vi "Host_Main.vi"() -> ()   [LabVIEW 2016]
uses:
  Typedefs/IO Lines State.ctl
  Typedefs/IO Lines Enable.ctl
  Typedefs/Truncate Waveform Settings.ctl
  Typedefs/Monitor Data Operation.ctl
  Typedefs/Host Cluster.ctl
  Typedefs/LV2G Operation.ctl
  <vilib>/NI/AMC/Read Termination Message.vi
  <vilib>/NI/AMC/Create Single Message.vi
  <vilib>/NI/AMC/Update Message Routing Info.vi
  <vilib>/NI/AMC/Globals.vi
  <vilib>/NI/AMC/Send Message.vi
  <vilib>/NI/AMC/AMC.lvlib
panel:
  in  "Tab Control":enum32{"Pattern", "Instruction"}(tab)
  out "Read Digital Waveform Graph":digitalwaveform(graph)
  in  "Truncate Waveform Settings":T1 {"End Idle Time(us)" format="%#.2f"; "Start Idle Time(us)" format="%#.2f"}
  out "Elapsed Time(ms)":u32 max=42
  in  "Monitor Time(ms)":u32 max=42000
  in  "IO Lines Read  Enable":T2={"Enable"=[FALSE, FALSE, FALSE, FALSE, FALSE, FALSE, FALSE, FALSE, FALSE, FALSE, FALSE, FALSE, FALSE, FALSE, FALSE, FALSE, FALSE, FALSE, FALSE, FALSE, FALSE, FALSE, FALSE, FALSE, FALSE, FALSE, FALSE, FALSE, FALSE, FALSE, FALSE, FALSE]}
  in  "Exit":bool
  in  "IO Lines Write  Enable":T2={"Enable"=[FALSE, FALSE, FALSE, FALSE, FALSE, FALSE, FALSE, FALSE, FALSE, FALSE, FALSE, FALSE, FALSE, FALSE, FALSE, FALSE, FALSE, FALSE, FALSE, FALSE, FALSE, FALSE, FALSE, FALSE, FALSE, FALSE, FALSE, FALSE, FALSE, FALSE, FALSE, FALSE]}
  in  "Monitoring":bool
  in  "Write Pattern":bool
  out "Write Digital Waveform Graph":digitalwaveform(graph)
  in  "IO Lines Pattteen":T3[](array[typedef]) {"Duration (us)" min=0.005 max=42550000.0 step=0.005 format="%#.3f"}
  # "Generator Settings"
  # "Monitor Settings"
  # "Duration(us)"
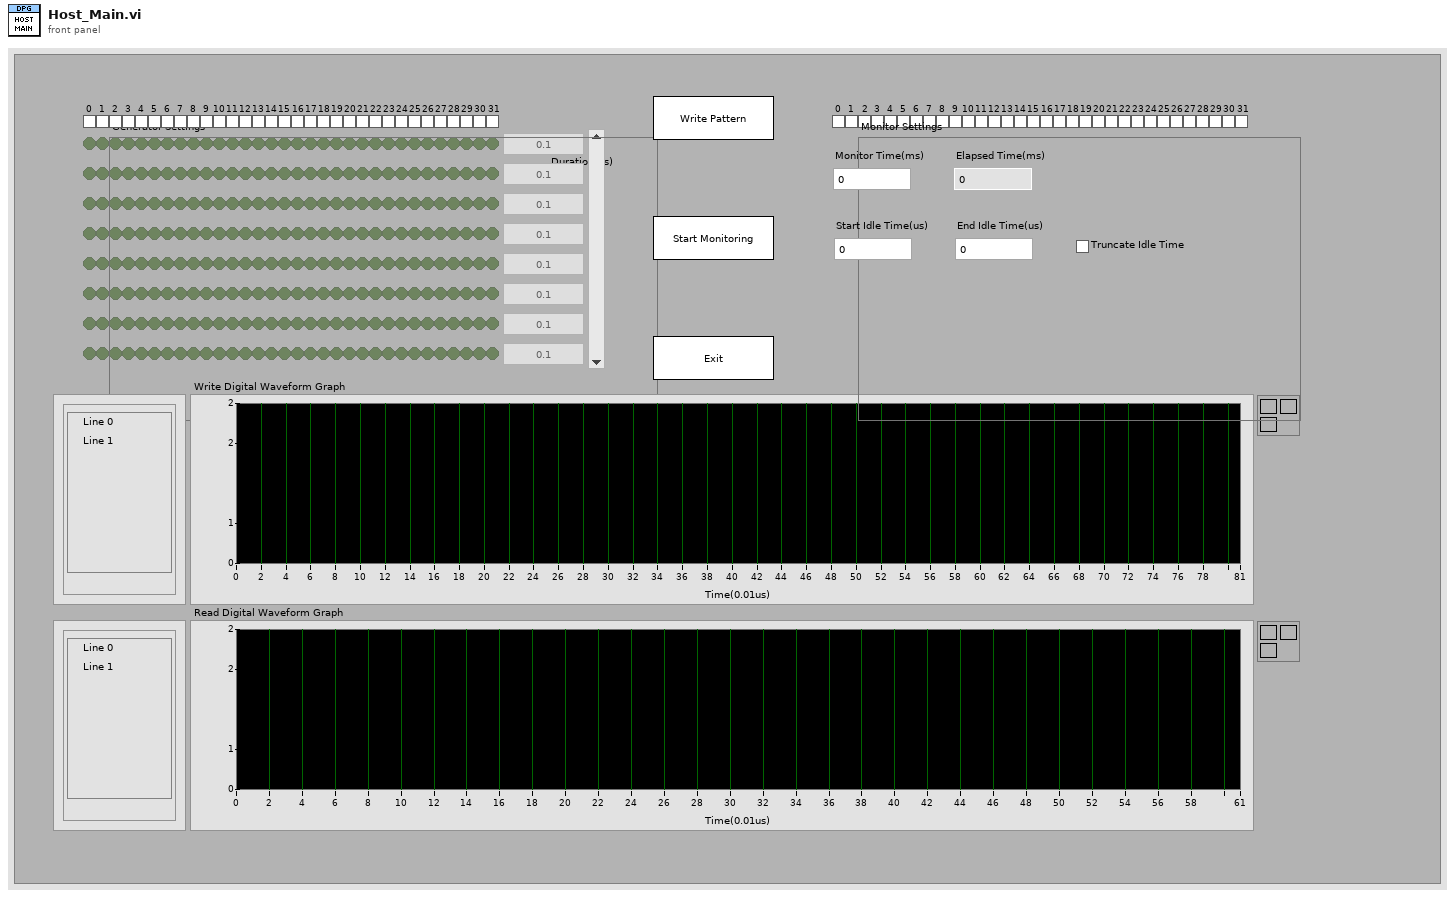
[diagram p1: front panel]
types:
  T1 = typedef "Truncate Waveform Settings.ctl" = cluster{"Truncate Idle Time":bool, "Start Idle Time(us)":dbl, "End Idle Time(us)":dbl}
  T2 = typedef "IO Lines Enable.ctl" = cluster{"Enable":bool[]}
  T3 = typedef "IO Lines State.ctl" = cluster{"State":bool[], "Duration (us)":dbl}
  T4 = typedef "AMC.lvlib/Message Queue.ctl" = refnum<queue>
  T5 = typedef "Monitor Data Operation.ctl" = enum16{"Obtain", "Enqueue", "Read Elements", "Flush", "Release", "Read Last Element"}
  T6 = typedef "Monitor Data Element.ctl" = cluster{"Pin Data":u32, "Transition ":u32}
  T7 = typedef "Host Cluster.ctl" = cluster{"Monitor Enable?":bool, "Start Time(ms)":u32}
  T8 = typedef "LV2G Operation.ctl" = enum16{"Initialize", "Set", "Get", "Close"}
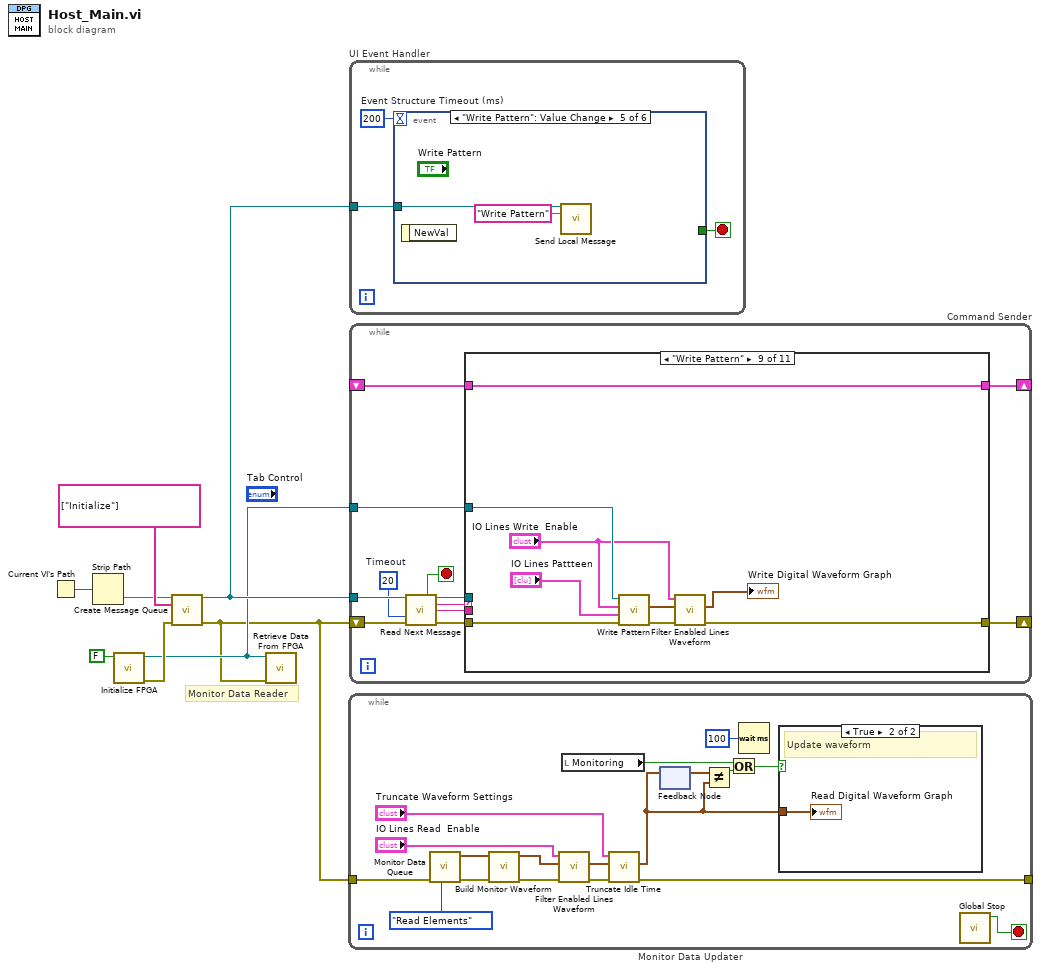
[diagram p0: block diagram]
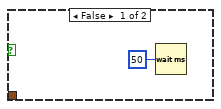
[diagram p2: hidden frame]
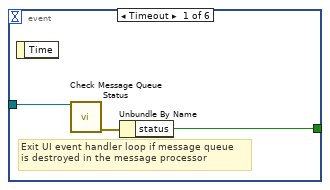
[diagram p3: hidden frame]
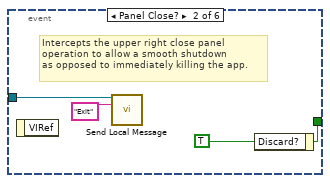
[diagram p4: hidden frame]
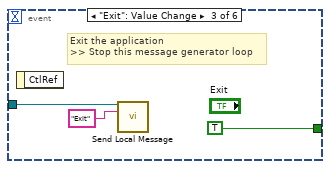
[diagram p5: hidden frame]
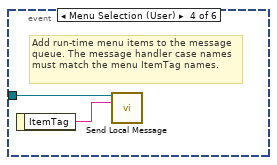
[diagram p6: hidden frame]
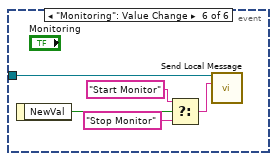
[diagram p7: hidden frame]
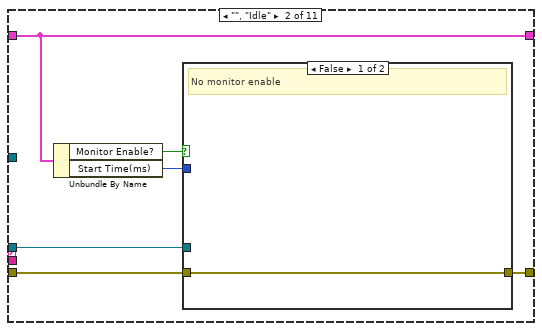
[diagram p9: hidden frame]
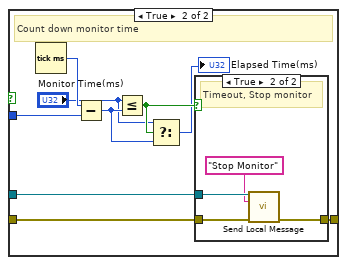
[diagram p10: hidden frame]
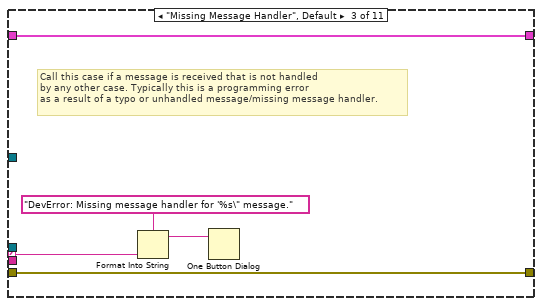
[diagram p12: hidden frame]
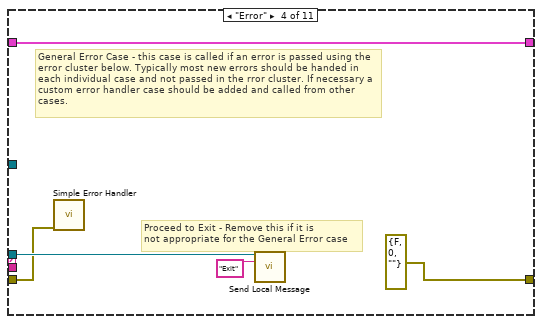
[diagram p13: hidden frame]
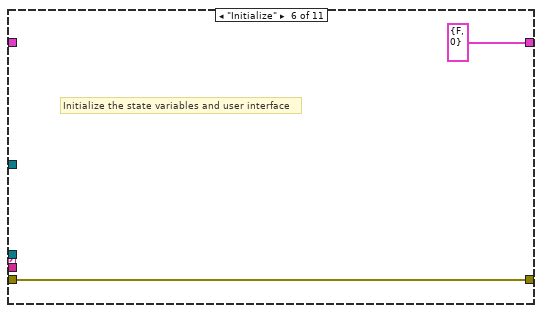
[diagram p15: hidden frame]
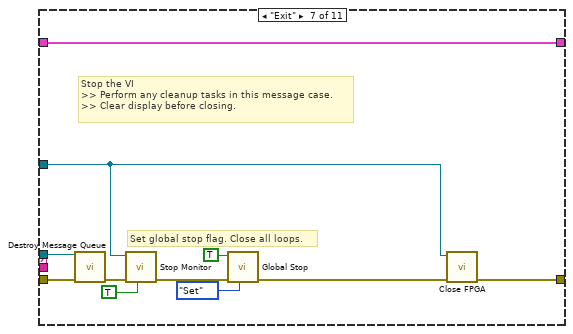
[diagram p16: hidden frame]
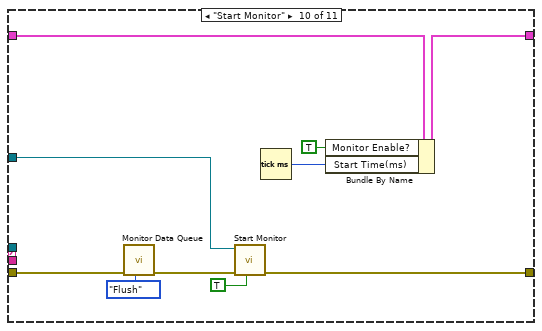
[diagram p18: hidden frame]
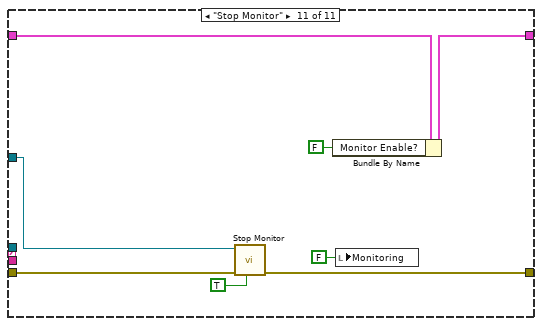
[diagram p19: hidden frame]
diagram:
  # "Monitor Data Reader"
  n1 = Current VI's Path() -> (path=w5:path)
  n2 = Strip Path(path=w5) -> (name=w7:string)  [unwired: 1 out]
  n3 = call "Initialize FPGA.vi"("Simulation?"=FALSE) -> ("error out"=w4:errorcluster, "FPGA VI Reference"=w3:refnum<k20>)  [unwired: 9 in]
  n4 = call <vilib>:"Create Message Queue.vi"("message queue name"=w7, "initial message names"=string[] ["Initialize"], "error in"=w4) -> ("message queue out"=w6:T4, "error out"=w2:errorcluster)  [unwired: 11 in]
  n5 = call "Retrieve Data From FPGA.vi"("error in (no error)"=w2, "FPGA VI Reference In"=w3) -> ()  [unwired: 9 in, 1 out]
  n6 = while "Monitor Data Updater" {
    tunnel: w2 -> [w26]
    tunnel: [w15] -> _
    stop <- w24 stop-if-true
    n7 = call "Monitor Data Queue.vi"("Queue Function"=Monitor_Data_Operation."Read Elements", "error in (no error)"=w26) -> ("error out"=w23:errorcluster, "Queue Elements"=w12:T6[])  [unwired: 6 in, 2 out]
    n8 = call "Build Monitor Waveform.vi"("error in (no error)"=w23, "Queue Elements"=w12) -> ("error out"=w22:errorcluster, "Digital Data Table"=w10:digitaldata)  [unwired: 8 in]
    n9 = call "Filter Enabled Lines Waveform.vi"("error in (no error)"=w22, "Pattern Digital Data"=w10, "IO Lines Enable"="IO Lines Read  Enable") -> ("error out"=w16:errorcluster, "Digital Waveform"=w14:digitalwaveform)  [unwired: 7 in]
    n10 = local read "Monitoring"() -> (w20:bool)
    n11 = call "Truncate Idle Time.vi"("error in (no error)"=w16, "Digital Waveform"=w14, "Truncate Waveform Settings"="Truncate Waveform Settings") -> ("error out"=w15:errorcluster, "Digital Waveform out"=w11:digitalwaveform)  [unwired: 7 in]
    n12 = feedback-in #1(w11) -> ()
    n13 = feedback #1() -> (w19:digitalwaveform)  [unwired: 1 in]
    n14 = Not Equal?(x=w19, y=w11) -> (x != y?=w17:bool)
    n15 = Or(x=w20, y=w17) -> (x .or. y?=w18:bool)
    n16 = Wait (ms)(milliseconds to wait=u32 100) -> ()  [unwired: 1 out]
    n17 = case shown="True" w18 {
      tunnel: w11 -> [_ w28]
      frame False {
        n18 = Wait (ms)(milliseconds to wait=u32 50) -> ()  [unwired: 1 out]
      }
      frame True {
        # "Update waveform"
        "Read Digital Waveform Graph" <- w28
      }
    }
    n19 = call "Global Stop.vi"() -> ("Stop? out"=w24:bool)  [unwired: 10 in, 1 out]
  }
  n20 = while "UI Event Handler" {
    tunnel: w6 -> [w29]
    stop <- w30 stop-if-true
    w31 = 200  # Event Structure Timeout (ms)
    n21 = event shown="[4] \"Write Pattern\": Value Change" {
      selector: _ -> [_ _ _ _ _ _]
      dyn-events: _ -> [_ _ _ _ _ _]
      timeout: w31 -> [_ _ _ _ _ _]
      tunnel: [w32 w37 TRUE ("Discard?") _ _ _] -> w30
      tunnel: w29 -> [w33 w35 w38 w41 w44 w49]
      event Timeout {
        # "Exit UI event handler loop if message queue\nis destroyed in the message processor"
        n22 = event-data() -> ()  [unwired: 2 out]
        n23 = call <vilib>:"Check Message Queue Status.vi"("message queue in"=w33) -> ("error out"=w34:errorcluster)  [unwired: 10 in, 4 out]
        n24 = Unbundle By Name(w34) -> ("status"=w32:bool)
      }
      event Panel Close? {
        w37 = TRUE ("Discard?")
        # "Intercepts the upper right close panel\noperation to allow a smooth shutdown\nas opposed to immediately killing the app."
        n25 = event-data() -> ()  [unwired: 2 out]
        n26 = call <vilib>:"Send Local Message.vi"("message queue in"=w35, "message name"="Exit") -> ()  [unwired: 11 in, 3 out]
        n27 = event-data("Discard?"=w37) -> ()  [unwired: 1 in, 1 out]
      }
      event "Exit": Value Change {
        # "Exit the application\n>> Stop this message generator loop"
        n28 = event-data() -> ()  [unwired: 2 out]
        n29 = call <vilib>:"Send Local Message.vi"("message queue in"=w38, "message name"="Exit") -> ()  [unwired: 11 in, 3 out]
      }
      event Menu Selection (User) {
        # "Add run-time menu items to the message\nqueue. The message handler case names must match the menu ItemTag names."
        n30 = event-data() -> ("ItemTag"=w42:string)  [unwired: 1 out]
        n31 = call <vilib>:"Send Local Message.vi"("message queue in"=w41, "message name"=w42) -> ()  [unwired: 11 in, 3 out]
      }
      event "Write Pattern": Value Change {
        n32 = event-data() -> ()  [unwired: 2 out]
        n33 = call <vilib>:"Send Local Message.vi"("message queue in"=w44, "message name"="Write Pattern") -> ()  [unwired: 11 in, 3 out]
      }
      event "Monitoring": Value Change {
        n34 = event-data() -> ("NewVal"=w47:bool)  [unwired: 1 out]
        n35 = Select(t="Start Monitor" ("message name"), s=w47, f="Stop Monitor") -> (s? t:f=w46:string)
        n36 = call <vilib>:"Send Local Message.vi"("message queue in"=w49, "message name"=w46) -> ()  [unwired: 11 in, 3 out]
      }
    }
  }
  n37 = while "Command Sender" {
    shift-left: w2 -> [w55]
    shift-right: [w59] -> _
    tunnel: w6 -> [w56]
    shift-left: _ -> [w61]
    shift-right: [w60] -> _
    tunnel: w3 -> [w50]
    stop <- w58 stop-if-true
    w51 = 20  # Timeout
    n38 = call <vilib>:"Read Next Message.vi"("message queue in"=w56, "timeout (1 ms)"=w51, "error in"=w55) -> ("exit process?"=w58:bool, "message queue out"=w57:T4, "message name"=w53:string, "message value"=w52:string, "error out"=w54:errorcluster)  [unwired: 5 in, 3 out]
    n39 = case shown="\"Write Pattern\"" w53 {
      selector: w53 -> [_ _ w87 _ _ _ _ _ _ _ _]
      tunnel: [w63 w69 w89 w94 w96 T7 {"Monitor Enable?"=FALSE, "Start Time(ms)"=0} ("state variables") w109 w111 w120 w123 w132] -> w60
      tunnel: w61 -> [w63 w69 w89 w94 w96 _ w109 w111 w120 w130 w138]
      tunnel: w57 -> [_ w66 _ w92 _ _ w107 _ _ _ _]
      tunnel: w54 -> [w62 w65 w88 w90 w95 w98 w108 w110 w117 w126 w137]
      tunnel: [w62 w64 w88 errorcluster {"status"=FALSE, "code"=0, "source"=""} ("error out") w95 w98 w99 w110 w112 w129 w136] -> w59
      tunnel: w52 -> [_ _ _ _ _ _ _ _ _ _ _]
      tunnel: w50 -> [_ _ _ _ _ _ w101 _ w119 w127 w134]
      frame "---------- Framework Operations ----------" {
        # "Dummy case to add a seperator in the Case Structure menu"
      }
      frame "", "Idle" {
        n40 = Unbundle By Name(w69) -> ("Monitor Enable?"=w68:bool, "Start Time(ms)"=w67:u32)
        n41 = case shown="False" w68 {
          tunnel: w67 -> [_ w78]
          tunnel: w66 -> [_ w77]
          tunnel: w65 -> [w70 w76]
          tunnel: [w70 w75] -> w64
          frame False {
            # "No monitor enable"
          }
          frame True {
            # "Count down monitor time"
            n42 = Tick Count (ms)() -> (millisecond timer value=w79:u32)
            n43 = Subtract(x=w79, y=w78) -> (x-y=w72:u32)
            n44 = Less Or Equal?(x="Monitor Time(ms)", y=w72) -> (x <= y?=w74:bool)
            n45 = Select(t="Monitor Time(ms)", s=w74, f=w72) -> (s? t:f=→"Elapsed Time(ms)":u32)
            n46 = case shown="True" w74 {
              tunnel: w77 -> [_ w84]
              tunnel: w76 -> [w80 w83]
              tunnel: [w80 w82] -> w75
              frame False {
                # "Continue"
              }
              frame True {
                # "Timeout, Stop monitor"
                n47 = call <vilib>:"Send Local Message.vi"("message queue in"=w84, "message name"="Stop Monitor", "error in"=w83) -> ("error out"=w82:errorcluster)  [unwired: 10 in, 2 out]
              }
            }
          }
        }
      }
      frame "Missing Message Handler", Default {
        # "Call this case if a message is received that is not handled \nby any other case. Typically this is a programming error\nas a result of a typo or unhandled message/missing message handler."
        n48 = Format Into String(format string="DevError: Missing message handler for '%s\" message." ("message"), w87) -> (resulting string=w85:string)  [unwired: 2 in, 1 out]
        n49 = One Button Dialog(message=w85) -> ()  [unwired: 2 out]
      }
      frame "Error" {
        # "Proceed to Exit - Remove this if it is\nnot appropriate for the General Error case"
        # "General Error Case - this case is called if an error is passed using the error cluster below. Typically most new errors should be handed in each individual case and not passed in the rror cluster. If necessary a custom error handler case should be added and called from other cases."
        n50 = call <vilib>:"Simple Error Handler.vi"("error in (no error)"=w90) -> ()  [unwired: 1 in, 8 out]
        n51 = call <vilib>:"Send Local Message.vi"("message queue in"=w92, "message name"="Exit") -> ()  [unwired: 11 in, 3 out]
      }
      frame "---------- Generic Operations ----------" {
        # "Dummy case to add a seperator in the Case Structure menu"
      }
      frame "Initialize" {
        # "Initialize the state variables and user interface"
      }
      frame "Exit" {
        # "Set global stop flag. Close all loops."
        # "Stop the VI\n>> Perform any cleanup tasks in this message case.\n>> Clear display before closing."
        n52 = call <vilib>:"Destroy Message Queue.vi"("message queue in"=w107, "error in"=w108) -> ("error out"=w104:errorcluster)  [unwired: 11 in, 2 out]
        n53 = call "Stop Monitor.vi"("Write to FPGA(T)"=TRUE, "error in (no error)"=w104, "FPGA VI Reference In"=w101) -> ("error out"=w103:errorcluster)  [unwired: 7 in, 1 out]
        n54 = call "Global Stop.vi"("Stop Operation (Get)"=LV2G_Operation."Set", "error in (no error)"=w103, "Stop?"=TRUE) -> ("error out"=w100:errorcluster)  [unwired: 7 in, 1 out]
        n55 = call "Close FPGA.vi"("error in (no error)"=w100, "Refnum in"=w101) -> ("error out"=w99:errorcluster)  [unwired: 9 in]
      }
      frame "---------- Application Operations ----------" {
        # "Dummy case to add a seperator in the Case Structure menu"
      }
      frame "Write Pattern" {
        n56 = call "Write Pattern.vi"("error in (no error)"=w117, "IO Lines Pattteen"="IO Lines Pattteen", "IO Lines Enable"="IO Lines Write  Enable", "Refnum in"=w119) -> ("error out"=w115:errorcluster, "Pattern Digital Data"=w116:digitaldata)  [unwired: 5 in, 1 out]
        n57 = call "Filter Enabled Lines Waveform.vi"("error in (no error)"=w115, "Pattern Digital Data"=w116, "IO Lines Enable"="IO Lines Write  Enable") -> ("error out"=w112:errorcluster, "Digital Waveform"=→"Write Digital Waveform Graph":digitalwaveform)  [unwired: 7 in]
      }
      frame "Start Monitor" {
        n58 = call "Monitor Data Queue.vi"("Queue Function"=Monitor_Data_Operation."Flush", "error in (no error)"=w126) -> ("error out"=w125:errorcluster)  [unwired: 6 in, 3 out]
        n59 = call "Start Monitor.vi"("Write to FPGA(T)"=TRUE, "error in (no error)"=w125, "FPGA VI Reference In"=w127) -> ("error out"=w129:errorcluster)  [unwired: 7 in, 1 out]
        n60 = Tick Count (ms)() -> (millisecond timer value=w121:u32)
        n61 = Bundle By Name(cluster=w130, "Monitor Enable?"=TRUE, "Start Time(ms)"=w121) -> (w123:T7)
      }
      frame "Stop Monitor" {
        n62 = call "Stop Monitor.vi"("Write to FPGA(T)"=TRUE, "error in (no error)"=w137, "FPGA VI Reference In"=w134) -> ("error out"=w136:errorcluster)  [unwired: 7 in, 1 out]
        n63 = Bundle By Name(cluster=w138, "Monitor Enable?"=FALSE) -> (w132:T7)
        n64 = local write "Monitoring"(FALSE ("Monitoring")) -> ()
      }
    }
  }
